vi "error-cluster2.vi"() -> ()   [LabVIEW 2011]
panel:
  out "String":string
  out "Boolean":bool
  out "error out":errorcluster
  in  "error in (no error)":errorcluster
  in  "Min Temp":dbl
  in  "Mx Temp":dbl
  in  "Current Temp":dbl
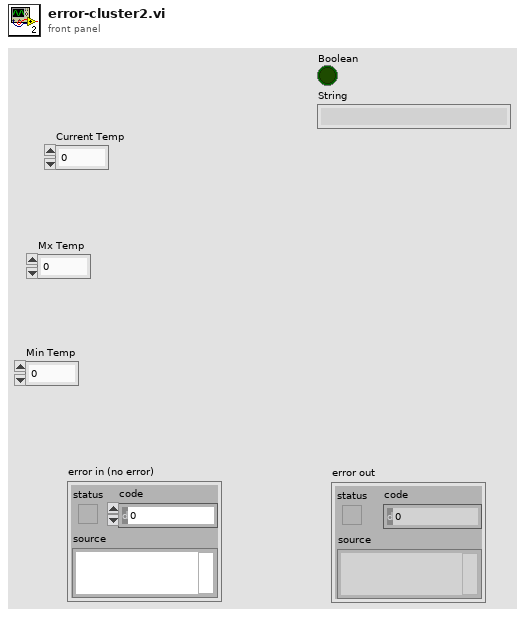
[diagram p1: front panel]
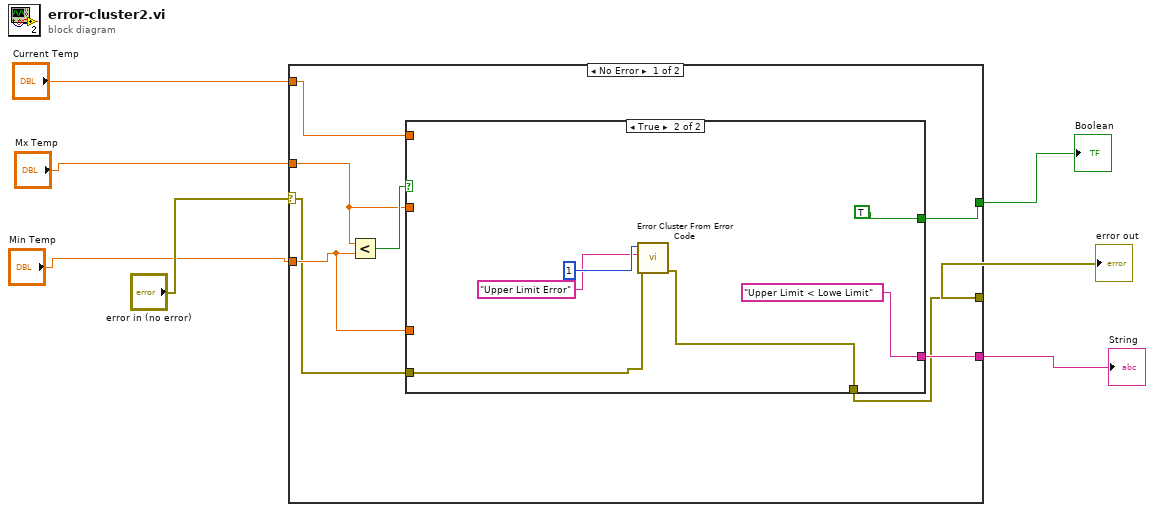
[diagram p0: block diagram]
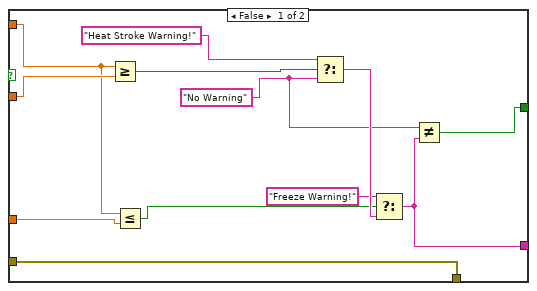
[diagram p2: hidden frame]
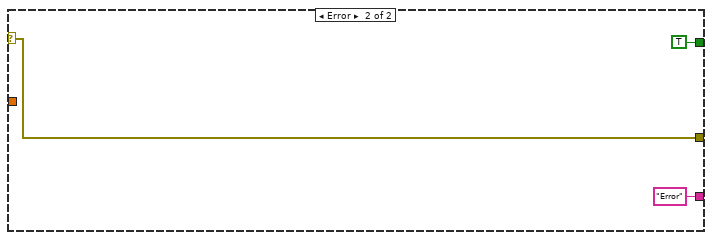
[diagram p3: hidden frame]
diagram:
  n1 = case shown="No Error" "error in (no error)" {
    selector: "error in (no error)" -> [w9 w36]
    tunnel: [w8 w36] -> w6
    tunnel: "Current Temp" -> [w15 _]
    tunnel: "Mx Temp" -> [w13 _]
    tunnel: "Min Temp" -> [w12 _]
    tunnel: [w11 TRUE] -> w2
    tunnel: [w10 "Error" ("t")] -> w1
    frame No Error {
      n2 = Less?(x=w13, y=w12) -> (x < y?=w14:bool)
      n3 = case shown="True" w14 {
        tunnel: w15 -> [w23 _]
        tunnel: w13 -> [w27 _]
        tunnel: w12 -> [w22 _]
        tunnel: [w18 TRUE] -> w11
        tunnel: [w17 "Upper Limit < Lowe Limit"] -> w10
        tunnel: w9 -> [w16 w29]
        tunnel: [w16 w28] -> w8
        frame False {
          w19 = "No Warning"
          n4 = Greater Or Equal?(x=w23, y=w27) -> (x >= y?=w26:bool)
          n5 = Less Or Equal?(x=w23, y=w22) -> (x <= y?=w21:bool)
          n6 = Select(t="Heat Stroke Warning!", s=w26, f=w19) -> (s? t:f=w24:string)
          n7 = Select(t="Freeze Warning!", s=w21, f=w24) -> (s? t:f=w17:string)
          n8 = Not Equal?(x=w19, y=w17) -> (x != y?=w18:bool)
        }
        frame True {
          n9 = call <vilib>:"Error Cluster From Error Code.vi"("error in (no error)"=w29, "error message (\"\")"="Upper Limit Error" ("error message (\"\")"), "error code (0)"=1) -> ("error out"=w28:errorcluster)  [unwired: 6 in]
        }
      }
    }
    frame Error {
    }
  }
  "error out" <- w6
  "Boolean" <- w2
  "String" <- w1
